vi "Zeroed Rotation Matrix.vi"(2 "Reference index":i32, 3 "Unreferenced Rotation Matrix":dbl[][](array[numeric]) format="%.2f") -> (1 "Referenced Rotation Matrix":dbl[][](graph))   [LabVIEW 2013]
panel:
  # "Copyright Americo A. Migliaccio (c) 2002 All Rights Reserved by Author"
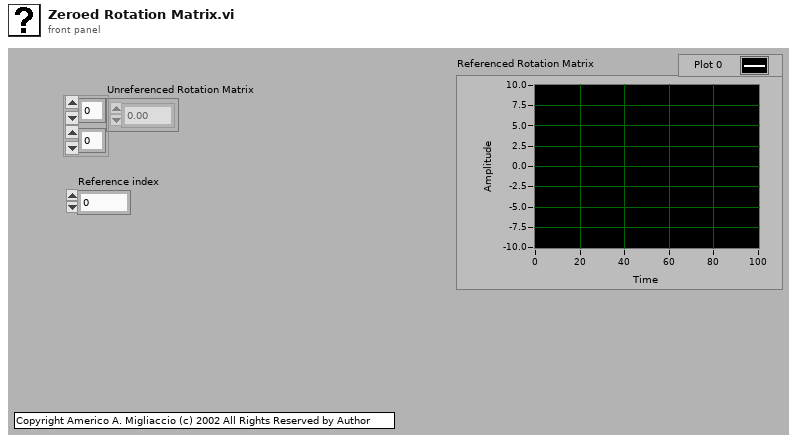
[diagram p1: front panel]
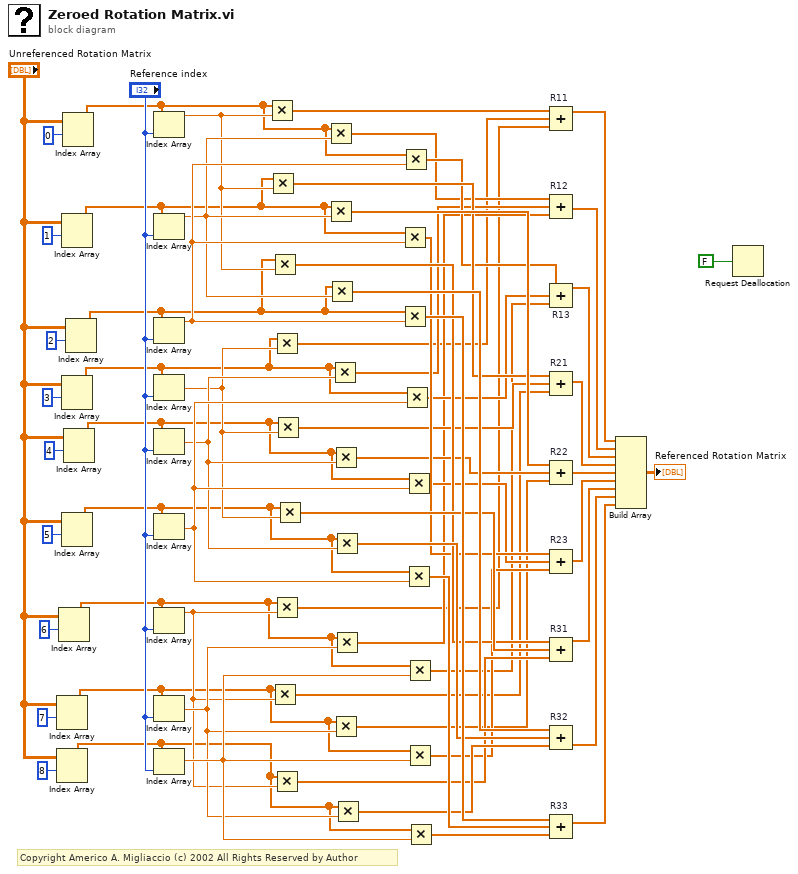
[diagram p0: block diagram]
diagram:
  # "Copyright Americo A. Migliaccio (c) 2002 All Rights Reserved by Author"
  n1 = Index Array(array="Unreferenced Rotation Matrix", index (row)=7 ("Index (row)")) -> (element=w13:dbl[])  [unwired: 1 in]
  n2 = Index Array(array="Unreferenced Rotation Matrix", index (row)=8 ("Index (row)")) -> (element=w12:dbl[])  [unwired: 1 in]
  n3 = Index Array(array="Unreferenced Rotation Matrix", index (row)=6 ("Index (row)")) -> (element=w14:dbl[])  [unwired: 1 in]
  n4 = Index Array(array="Unreferenced Rotation Matrix", index (row)=1 ("Index (row)")) -> (element=w19:dbl[])  [unwired: 1 in]
  n5 = Index Array(array="Unreferenced Rotation Matrix", index (row)=3 ("Index (row)")) -> (element=w17:dbl[])  [unwired: 1 in]
  n6 = Index Array(array="Unreferenced Rotation Matrix", index (row)=5 ("Index (row)")) -> (element=w15:dbl[])  [unwired: 1 in]
  n7 = Index Array(array="Unreferenced Rotation Matrix", index (row)=0 ("Disabled Index (col)")) -> (element=w20:dbl[])  [unwired: 1 in]
  n8 = Index Array(array="Unreferenced Rotation Matrix", index (row)=4 ("Index (row)")) -> (element=w16:dbl[])  [unwired: 1 in]
  n9 = Index Array(array="Unreferenced Rotation Matrix", index (row)=2 ("Index (row)")) -> (element=w18:dbl[])  [unwired: 1 in]
  n10 = Index Array(array=w20, index="Reference index") -> (element=w41:dbl)
  n11 = Index Array(array=w19, index="Reference index") -> (element=w46:dbl)
  n12 = Index Array(array=w18, index="Reference index") -> (element=w53:dbl)
  n13 = Index Array(array=w17, index="Reference index") -> (element=w43:dbl)
  n14 = Index Array(array=w16, index="Reference index") -> (element=w48:dbl)
  n15 = Index Array(array=w15, index="Reference index") -> (element=w55:dbl)
  n16 = Index Array(array=w14, index="Reference index") -> (element=w50:dbl)
  n17 = Index Array(array=w13, index="Reference index") -> (element=w51:dbl)
  n18 = Index Array(array=w12, index="Reference index") -> (element=w57:dbl)
  n19 = Multiply(x=w20, y=w41) -> (x*y=w23:dbl[])
  n20 = Multiply(x=w19, y=w41) -> (x*y=w32:dbl[])
  n21 = Multiply(x=w18, y=w41) -> (x*y=w42:dbl[])
  n22 = Multiply(x=w13, y=w50) -> (x*y=w34:dbl[])
  n23 = Multiply(x=w17, y=w43) -> (x*y=w24:dbl[])
  n24 = Multiply(x=w14, y=w50) -> (x*y=w25:dbl[])
  n25 = Multiply(x=w12, y=w50) -> (x*y=w45:dbl[])
  n26 = Multiply(x=w16, y=w43) -> (x*y=w33:dbl[])
  n27 = Multiply(x=w15, y=w43) -> (x*y=w44:dbl[])
  n28 = Multiply(x=w20, y=w46) -> (x*y=w26:dbl[])
  n29 = Multiply(x=w19, y=w46) -> (x*y=w37:dbl[])
  n30 = Multiply(x=w18, y=w46) -> (x*y=w47:dbl[])
  n31 = Multiply(x=w17, y=w48) -> (x*y=w27:dbl[])
  n32 = Multiply(x=w16, y=w48) -> (x*y=w36:dbl[])
  n33 = Multiply(x=w13, y=w51) -> (x*y=w35:dbl[])
  n34 = Multiply(x=w15, y=w48) -> (x*y=w49:dbl[])
  n35 = Multiply(x=w14, y=w51) -> (x*y=w28:dbl[])
  n36 = Multiply(x=w12, y=w51) -> (x*y=w52:dbl[])
  n37 = Multiply(x=w19, y=w53) -> (x*y=w40:dbl[])
  n38 = Multiply(x=w18, y=w53) -> (x*y=w54:dbl[])
  n39 = Multiply(x=w20, y=w53) -> (x*y=w29:dbl[])
  n40 = Multiply(x=w17, y=w55) -> (x*y=w30:dbl[])
  n41 = Multiply(x=w16, y=w55) -> (x*y=w38:dbl[])
  n42 = Multiply(x=w15, y=w55) -> (x*y=w56:dbl[])
  n43 = Multiply(x=w14, y=w57) -> (x*y=w31:dbl[])
  n44 = Multiply(x=w13, y=w57) -> (x*y=w39:dbl[])
  n45 = Multiply(x=w12, y=w57) -> (x*y=w58:dbl[])
  n46 = Compound Arithmetic op=ADD "R11"(w23, w24, w25) -> (w59:dbl[])
  n47 = Compound Arithmetic op=ADD "R12"(w26, w27, w28) -> (w60:dbl[])
  n48 = Compound Arithmetic op=ADD "R13"(w29, w30, w31) -> (w61:dbl[])
  n49 = Compound Arithmetic op=ADD "R21"(w32, w33, w34) -> (w62:dbl[])
  n50 = Compound Arithmetic op=ADD "R22"(w37, w36, w35) -> (w63:dbl[])
  n51 = Compound Arithmetic op=ADD "R23"(w40, w38, w39) -> (w64:dbl[])
  n52 = Compound Arithmetic op=ADD "R31"(w42, w44, w45) -> (w65:dbl[])
  n53 = Compound Arithmetic op=ADD "R32"(w47, w49, w52) -> (w66:dbl[])
  n54 = Compound Arithmetic op=ADD "R33"(w54, w56, w58) -> (w67:dbl[])
  n55 = Build Array(w59, w60, w61, w62, w63, w64, w65, w66, w67) -> (→"Referenced Rotation Matrix":dbl[][])
  n56 = Request Deallocation(FALSE ("flag")) -> ()
